vi "Update Test Sequence Table.vi"(8 "Listbox Reference":refnum<vi>, 10 "Test Sequence":T1[](array[typedef]), 11 "Valid?":bool) -> ()   [LabVIEW 2015]
uses:
  Single Test Sequence.ctl
  Test Sequence Action.ctl
  Valve Action Enum.ctl
  Valve Name Enum.ctl
  Test Sequence Trigger.ctl
  Sensors/Sensor Enum.ctl
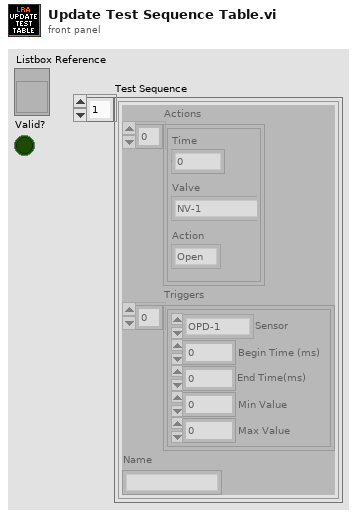
[diagram p1: front panel]
types:
  T1 = typedef "Single Test Sequence.ctl" = cluster{"Actions":T2[], "Triggers":T5[], "Name":string}
  T2 = typedef "Test Sequence Action.ctl" = cluster{"Time":i32, "Action":T3, "Valve":T4}
  T3 = typedef "Valve Action Enum.ctl" = enum16{"Open", "Close"}
  T4 = typedef "Valve Name Enum.ctl" = enum16{"NV-1", "NV-2", "OV-2", "OV-3", "OV-4", "WV-2"}
  T5 = typedef "Test Sequence Trigger.ctl" = cluster{"Sensor":T6, "Begin Time (ms)":dbl, "End Time(ms)":dbl, "Min Value":dbl, "Max Value":dbl}
  T6 = typedef "Sensor Enum.ctl" = enum16{"OPD-1", "OPD-2", "OPD-3", "OTC-1", ""}
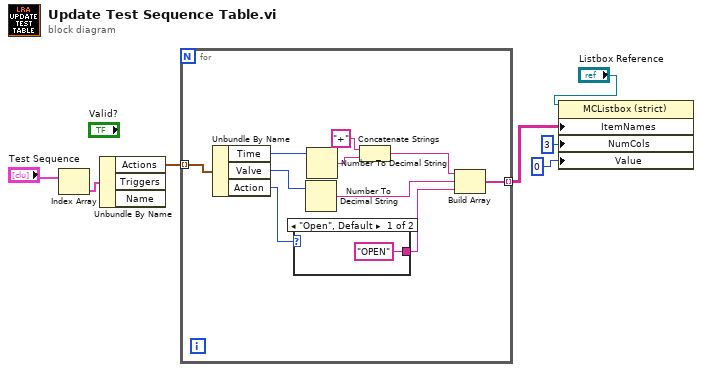
[diagram p0: block diagram]
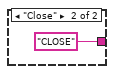
[diagram p2: hidden frame]
diagram:
  n1 = Index Array(array="Test Sequence") -> (element=w2:T1)  [unwired: 1 in]
  n2 = Unbundle By Name(w2) -> ("Actions"=w1:T2[])  [unwired: 2 out]
  n3 = for {
    tunnel: [w13] -> w5 mode=indexing
    tunnel: w1 -> [w12] mode=indexing
    n4 = Unbundle By Name(w12) -> ("Time"=w9:i32, "Valve"=w10:T4, "Action"=w11:T3)
    n5 = case shown="\"Open\", Default" w11 {
      tunnel: ["OPEN" "CLOSE"] -> w14
      frame "Open", Default {
      }
      frame "Close" {
      }
    }
    n6 = Number To Decimal String(number=w10) -> (decimal integer string=w15:string)  [unwired: 1 in]
    n7 = Number To Decimal String(number=w9) -> (decimal integer string=w8:string)  [unwired: 1 in]
    n8 = Concatenate Strings("+" ("string"), w8) -> (w16:string)
    n9 = Build Array(w16, w15, w14) -> (w13:string[])
  }
  n10 = property class="MCListbox (strict)"(reference="Listbox Reference", "ItemNames"=w5, "NumCols"=u32 3 ("Number of Columns"), "Value"=0 ("Focus Row")) -> ()  [unwired: 1 in, 2 out]
